vi "ARRAY INPX TO SCRIPT RTS .vi"(11 "TDX":bool[](array[boolean])) -> (3 "SCRIPT OUT":string[](array[string]))   [LabVIEW 2014]
uses:
  CAP-USB.lvlib
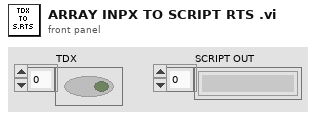
[diagram p1: front panel]
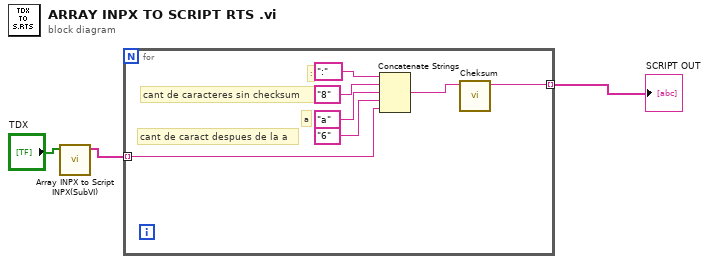
[diagram p0: block diagram]
diagram:
  n1 = call "Array INPX to Script INPX(SubVI).vi"("INPX IN"="TDX") -> ("INPX CONFIG"=w1:string[])  [unwired: 10 in]
  n2 = for {
    tunnel: w1 -> [w6] mode=indexing
    tunnel: [w4] -> w3 mode=indexing
    # "cant de caract despues de la a"
    # "a"
    # "cant de caracteres sin checksum"
    # ":"
    n3 = Concatenate Strings(":" ("string"), "8" ("string"), "a" ("string"), "6" ("string"), w6) -> (w5:string)
    n4 = call "Cheksum.vi"("Trama IN"=w5) -> ("Trama RTS"=w4:string)  [unwired: 10 in]
  }
  "SCRIPT OUT" <- w3
